vi "Stop motor -- subVI.vi"(8 "error in (no error)":errorcluster, 11 "VISA Refnum in":refnum<visa-resource-name>) -> (0 "error out":errorcluster, 2 "read buffer 2":string, 3 "Position":i32)   [LabVIEW 2020, in "Arduino stepper.lvlib"]
uses:
  Arduino stepper.lvlib
  <vilib>/Instr/_visa.llb/VISA Flush IO Buffer Mask.ctl
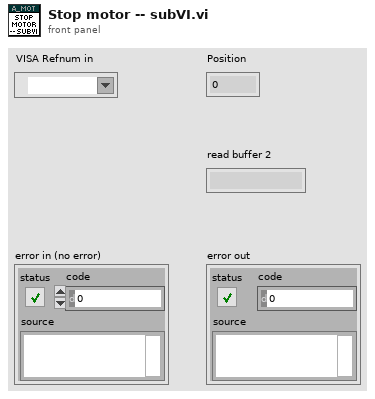
[diagram p1: front panel]
types:
  T1 = typedef "VISA Flush IO Buffer Mask.ctl" = u16
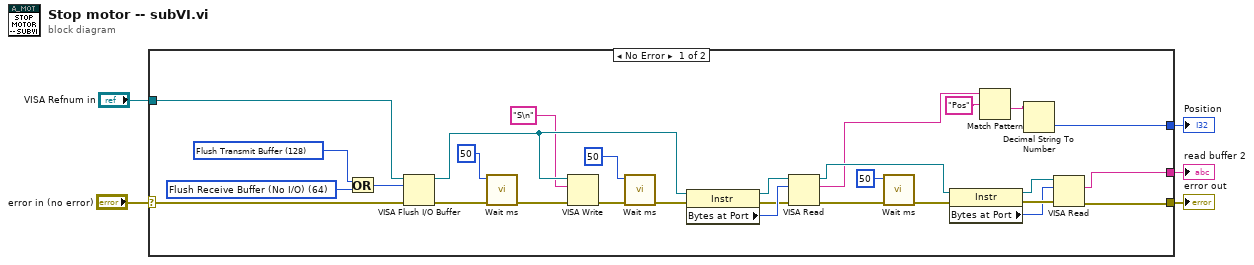
[diagram p0: block diagram]
diagram:
  n1 = case shown="No Error" "error in (no error)" {
    selector: "error in (no error)" -> [w22 w35]
    tunnel: "VISA Refnum in" -> [w23 _]
    tunnel: [w21 w35] -> w3
    tunnel: [w16 _] -> w2
    tunnel: [w12 _] -> w1
    frame No Error {
      w7 = T1 64 items=["Flush Receive Buffer"=16, "Write Transmit Buffer to Device"=32, "Flush Receive Buffer (No I/O)"=64, "Flush Transmit Buffer"=128] ("y")
      w8 = T1 128 items=["Flush Receive Buffer"=16, "Write Transmit Buffer to Device"=32, "Flush Receive Buffer (No I/O)"=64, "Flush Transmit Buffer"=128] ("Mask")
      n2 = Or(x=w8, y=w7) -> (x .or. y?=w6:T1)
      n3 = VISA Flush I/O Buffer(VISA resource name=w23, mask (16)=w6, error in (no error)=w22) -> (VISA resource name out=w31:refnum<visa-resource-name>, error out=w24:errorcluster)
      n4 = call "Wait ms.vi"("error in (no error)"=w24, "milliseconds to wait"=u32 50) -> ("error out"=w26:errorcluster)  [unwired: 9 in]
      n5 = VISA Write(VISA resource name=w31, write buffer="S\n", error in (no error)=w26) -> (error out=w28:errorcluster)  [unwired: 2 out]
      n6 = call "Wait ms.vi"("error in (no error)"=w28, "milliseconds to wait"=u32 50) -> ("error out"=w30:errorcluster)  [unwired: 9 in]
      n7 = property class="Instr"(reference=w31, error in=w30) -> (reference out=w33:refnum<visa-resource-name>, error out=w32:errorcluster, "Bytes at Port"=w34:u32)
      n8 = VISA Read(VISA resource name=w33, byte count=w34, error in (no error)=w32) -> (VISA resource name out=w18:refnum<visa-resource-name>, read buffer=w13:string, error out=w11:errorcluster)  [unwired: 1 out]
      n9 = call "Wait ms.vi"("error in (no error)"=w11, "milliseconds to wait"=u32 50) -> ("error out"=w10:errorcluster)  [unwired: 9 in]
      n10 = property class="Instr"(reference=w18, error in=w10) -> (reference out=w17:refnum<visa-resource-name>, error out=w20:errorcluster, "Bytes at Port"=w19:u32)
      n11 = Match Pattern(string=w13, regular expression="Pos") -> (after substring=w14:string)  [unwired: 1 in, 3 out]
      n12 = Decimal String To Number(string=w14) -> (number=w12:i32)  [unwired: 2 in, 1 out]
      n13 = VISA Read(VISA resource name=w17, byte count=w19, error in (no error)=w20) -> (read buffer=w16:string, error out=w21:errorcluster)  [unwired: 2 out]
    }
    frame Error {
    }
  }
  "error out" <- w3
  "read buffer 2" <- w2
  "Position" <- w1
